vi "Analyze Data.vi"(0 "날씨 데이터":dynamicdata(waveform), 11 "에러 입력":errorcluster) -> (4 "시간":dbl, 6 "온도":dbl, 8 "풍속":dbl, 15 "에러 출력":errorcluster)   [LabVIEW 2010]
uses:
  Instance           1 20Saved   Analyze Data .vi
  Instance           3 20Saved   Analyze Data .vi
  Instance           4 20Saved   Analyze Data .vi
  Instance           5 20Saved   Analyze Data .vi
  Instance           2 20Saved   Analyze Data .vi
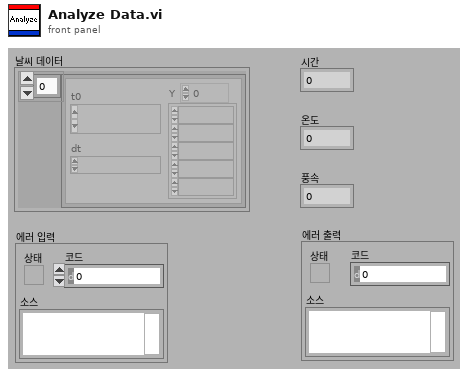
[diagram p1: front panel]
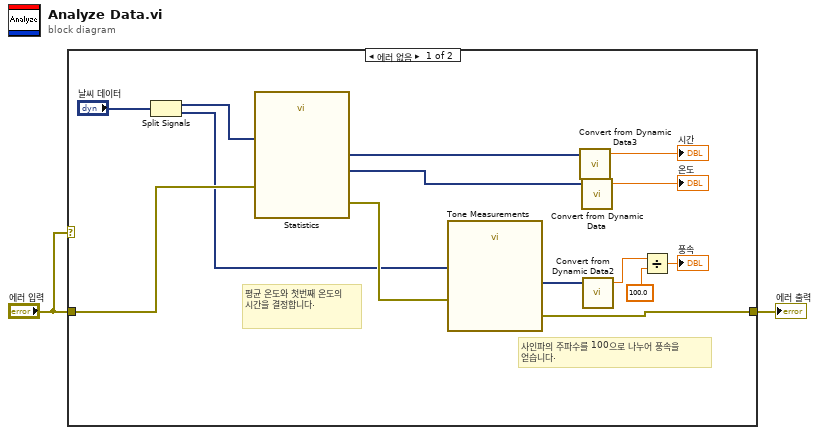
[diagram p0: block diagram]
diagram:
  n1 = case shown="에러 없음" "에러 입력" {
    tunnel: "에러 입력" -> [w16 w17]
    tunnel: [w10 w17] -> w2
    frame No Error {
      # "사인파의 주파수를 100으로 나누어 풍속을 얻습니다."
      # "평균 온도와 첫번째 온도의 시간을 결정합니다."
      n2 = Split Signals("날씨 데이터") -> (w4:dynamicdata, w3:dynamicdata)  [unwired: 2 in]
      n3 = call "Statistics"("Signals"=w4, "error in (no error)"=w16) -> ("Arithmetic Mean"=w5:dynamicdata, "First Time"=w11:dynamicdata, "error out"=w9:errorcluster)  [unwired: 23 in]
      n4 = call "Tone Measurements"("error in (no error)"=w9, "Signals"=w3) -> ("error out"=w10:errorcluster, "Frequency"=w7:dynamicdata)  [unwired: 8 in]
      n5 = call "Convert from Dynamic Data3"("Dynamic Data Type"=w11) -> ("Scalar"=→"시간":dbl)  [unwired: 3 in]
      n6 = call "Convert from Dynamic Data"("Dynamic Data Type"=w5) -> ("Scalar"=→"온도":dbl)  [unwired: 3 in]
      n7 = call "Convert from Dynamic Data2"("Dynamic Data Type"=w7) -> ("Scalar"=w8:dbl)  [unwired: 3 in]
      n8 = Divide(x=w8, y=100.0) -> (x/y=→"풍속":dbl)
    }
    frame Error {
    }
  }
  "에러 출력" <- w2
